vi "Drive Initialize.vi"(8 "Right Slave":u8, 9 "Right Master":u8, 10 "Left Slave":u8, 11 "Left Master":u8) -> (1 "RightMasterDevRef":T1, 3 "LeftMasterDevRef":T1)   [LabVIEW 2019]
uses:
  <vilib>/Rock Robotics/WPI/MotorControl/WPI_MotorControlDeviceRef.ctl
  <vilib>/Rock Robotics/WPI/MotorControl/WPI_MotorControlType.ctl
  <vilib>/Rock Robotics/SystemInterfaces/DIO/FPGA_DIOPWMChannel.ctl
  <vilib>/Rock Robotics/WPI/PWM/WPI_PWMDeadband.ctl
  <vilib>/Rock Robotics/SystemInterfaces/DIO/FPGA_DIOChannel.ctl
  <vilib>/Rock Robotics/WPI/ThirdParty/Phoenix-LabVIEW/Motor Controller/Controls/CTRE_Phoenix_MotorControl_NeutralMode.ctl
  .Team Code/Contants.vi
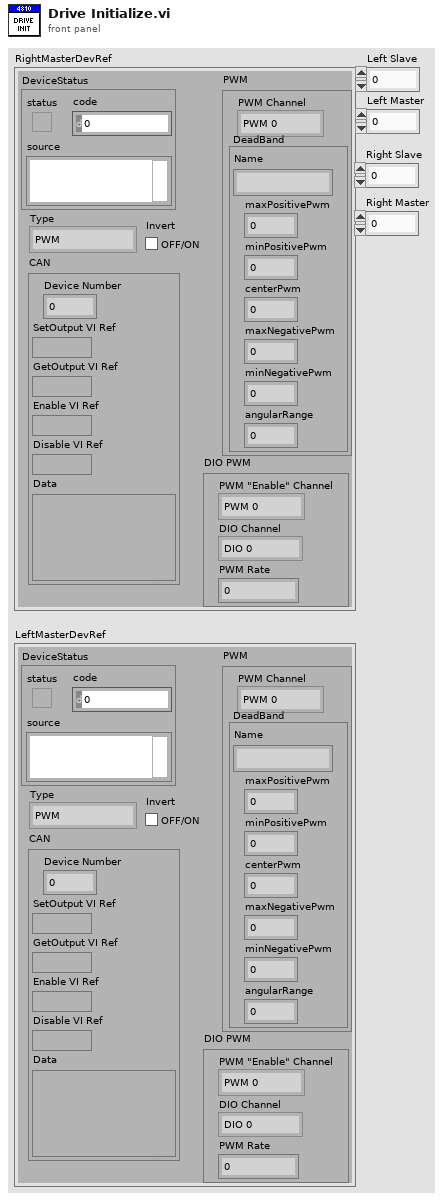
[diagram p1: front panel]
types:
  T1 = typedef "WPI_MotorControlDeviceRef.ctl" = cluster{"DeviceStatus":errorcluster, "Type":T2, "PWM":cluster{"PWM Channel":T3, "DeadBand":T4}, "CAN":cluster{"Device Number":u8, "SetOutput VI Ref":variant, "GetOutput VI Ref":variant, "Enable VI Ref":variant, "Disable VI Ref":variant, "Data":variant}, "Invert":bool, "DIO PWM":cluster{"PWM \"Enable\" Channel":T3, "DIOChannel":T5, "PWM Rate":dbl}}
  T2 = typedef "WPI_MotorControlType.ctl" = enum16{"PWM", "CAN", "DIO PWM"}
  T3 = typedef "FPGA_DIOPWMChannel.ctl" = enum8{"PWM 0", "PWM 1", "PWM 2", "PWM 3", "PWM 4", "PWM 5", "PWM 6", "PWM 7", "PWM 8", "PWM 9", "PWM MXP 0", "PWM MXP 1", "PWM MXP 2", "PWM MXP 3", "PWM MXP 4", "PWM MXP 5", "PWM MXP 6", "PWM MXP 7", "PWM MXP 8", "PWM MXP 9", "Invalid"}
  T4 = typedef "WPI_PWMDeadband.ctl" = cluster{"Name":string, "maxPositivePwm":i32, "minPositivePwm":i32, "centerPwm":i32, "maxNegativePwm":i32, "minNegativePwm":i32, "angularRange":u16}
  T5 = typedef "FPGA_DIOChannel.ctl" = enum8{"DIO 0", "DIO 1", "DIO 2", "DIO 3", "DIO 4", "DIO 5", "DIO 6", "DIO 7", "DIO 8", "DIO 9", "DIO MXP 0", "DIO MXP 1", "DIO MXP 2", "DIO MXP 3", "DIO MXP 4", "DIO MXP 5", "DIO MXP 6", "DIO MXP 7", "DIO MXP 8", "DIO MXP 9", "DIO MXP 10", "DIO MXP 11", "DIO MXP 12", "DIO MXP 13", "DIO MXP 14", "DIO MXP 15", "SPI Port CS1", "SPI Port CS2", "SPI Port CS3", "SPI Port MISO", "SPI Port MOSI", "Invalid"}
  T6 = typedef "CTRE_Phoenix_MotorControl_NeutralMode.ctl" = enum8{"EEPROMSetting", "Override to Coast", "Override to Brake"}
  T7 = cluster{"Cruise Velocity":i32, "Acceleration":i32}
  T8 = cluster{"P":dbl, "I":dbl, "D":dbl, "F":dbl, "I Zone":dbl}
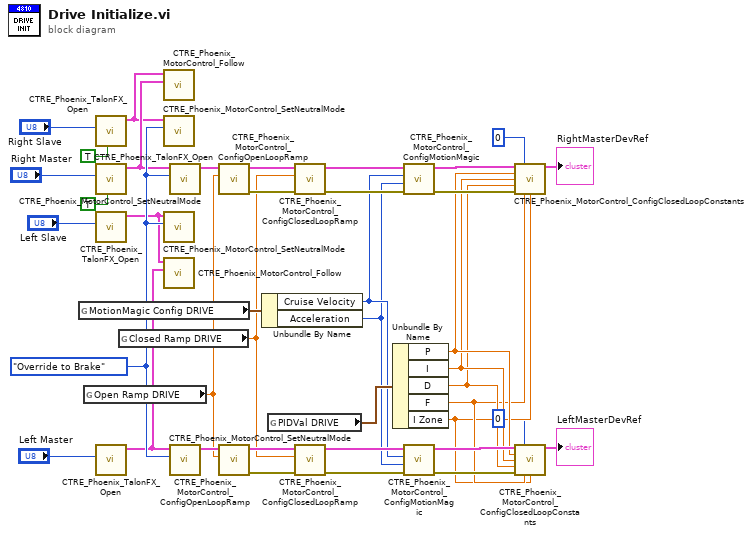
[diagram p0: block diagram]
diagram:
  w40 = CTRE_Phoenix_MotorControl_NeutralMode."Override to Brake" ("Motor Control Neutral Mode")
  n1 = global read "Contants.vi" "MotionMagic Config DRIVE"() -> (w15:T7)
  n2 = global read "Contants.vi" "Open Ramp DRIVE"() -> (w5:dbl)
  n3 = call <vilib>:"CTRE_Phoenix_TalonFX_Open.vi"("Invert"=TRUE, "Device Number"="Right Slave") -> ("CAN Talon SRX Ref"=w38:T1)  [unwired: 8 in, 1 out]
  n4 = call <vilib>:"CTRE_Phoenix_TalonFX_Open.vi"("Invert"=TRUE, "Device Number"="Right Master") -> ("CAN Talon SRX Ref"=w39:T1)  [unwired: 8 in, 1 out]
  n5 = call <vilib>:"CTRE_Phoenix_TalonFX_Open.vi"("Device Number"="Left Slave") -> ("CAN Talon SRX Ref"=w36:T1)  [unwired: 9 in, 1 out]
  n6 = call <vilib>:"CTRE_Phoenix_TalonFX_Open.vi"("Device Number"="Left Master") -> ("CAN Talon SRX Ref"=w37:T1)  [unwired: 9 in, 1 out]
  n7 = global read "Contants.vi" "Closed Ramp DRIVE"() -> (w6:dbl)
  n8 = call <vilib>:"CTRE_Phoenix_MotorControl_Follow.vi"("Master Controller to Follow"=w39, "PhoenixMotorControlDevRef"=w38) -> ()  [unwired: 8 in, 2 out]
  n9 = call <vilib>:"CTRE_Phoenix_MotorControl_SetNeutralMode.vi"("Motor Control Neutral Mode"=w40, "PhoenixMotorControlDevRef"=w38) -> ()  [unwired: 8 in, 2 out]
  n10 = call <vilib>:"CTRE_Phoenix_MotorControl_SetNeutralMode.vi"("Motor Control Neutral Mode"=w40, "PhoenixMotorControlDevRef"=w36) -> ()  [unwired: 8 in, 2 out]
  n11 = call <vilib>:"CTRE_Phoenix_MotorControl_Follow.vi"("Master Controller to Follow"=w37, "PhoenixMotorControlDevRef"=w36) -> ()  [unwired: 8 in, 2 out]
  n12 = call <vilib>:"CTRE_Phoenix_MotorControl_SetNeutralMode.vi"("Motor Control Neutral Mode"=w40, "PhoenixMotorControlDevRef"=w39) -> ("PhoenixMotorControlDevRef"=w17:T1)  [unwired: 8 in, 1 out]
  n13 = call <vilib>:"CTRE_Phoenix_MotorControl_SetNeutralMode.vi"("Motor Control Neutral Mode"=w40, "PhoenixMotorControlDevRef"=w37) -> ("PhoenixMotorControlDevRef"=w25:T1)  [unwired: 8 in, 1 out]
  n14 = call <vilib>:"CTRE_Phoenix_MotorControl_ConfigOpenLoopRamp.vi"("secondsFromNeutralToFull"=w5, "PhoenixMotorControlDevRef"=w17) -> ("error out"=w18:errorcluster, "PhoenixMotorControlDevRef"=w19:T1)  [unwired: 8 in]
  n15 = call <vilib>:"CTRE_Phoenix_MotorControl_ConfigOpenLoopRamp.vi"("secondsFromNeutralToFull"=w5, "PhoenixMotorControlDevRef"=w25) -> ("error out"=w31:errorcluster, "PhoenixMotorControlDevRef"=w30:T1)  [unwired: 8 in]
  n16 = Unbundle By Name(w15) -> ("Cruise Velocity"=w8:i32, "Acceleration"=w7:i32)
  n17 = global read "Contants.vi" "PIDVal DRIVE"() -> (w14:T8)
  n18 = call <vilib>:"CTRE_Phoenix_MotorControl_ConfigClosedLoopRamp.vi"("error in (no error)"=w18, "secondsFromNeutralToFull"=w6, "PhoenixMotorControlDevRef"=w19) -> ("error out"=w23:errorcluster, "PhoenixMotorControlDevRef"=w20:T1)  [unwired: 7 in]
  n19 = call <vilib>:"CTRE_Phoenix_MotorControl_ConfigClosedLoopRamp.vi"("error in (no error)"=w31, "secondsFromNeutralToFull"=w6, "PhoenixMotorControlDevRef"=w30) -> ("error out"=w26:errorcluster, "PhoenixMotorControlDevRef"=w29:T1)  [unwired: 7 in]
  n20 = Unbundle By Name(w14) -> ("P"=w13:dbl, "I"=w12:dbl, "D"=w11:dbl, "F"=w10:dbl, "I Zone"=w9:dbl)
  n21 = call <vilib>:"CTRE_Phoenix_MotorControl_ConfigMotionMagic.vi"("error in (no error)"=w23, "Acceleration"=w7, "Cruise Velocity"=w8, "PhoenixMotorControlDevRef"=w20) -> ("error out"=w22:errorcluster, "PhoenixMotorControlDevRef"=w21:T1)  [unwired: 6 in]
  n22 = call <vilib>:"CTRE_Phoenix_MotorControl_ConfigMotionMagic.vi"("error in (no error)"=w26, "Acceleration"=w7, "Cruise Velocity"=w8, "PhoenixMotorControlDevRef"=w29) -> ("error out"=w27:errorcluster, "PhoenixMotorControlDevRef"=w28:T1)  [unwired: 6 in]
  n23 = call <vilib>:"CTRE_Phoenix_MotorControl_ConfigClosedLoopConstants.vi"("PhoenixMotorControlDevRef"=w21, "slotIdx"=0, "P"=w13, "I"=w12, "D"=w11, "error in (no error)"=w22, "F"=w10, "I Zone"=w9) -> ("PhoenixMotorControlDevRef"=→"RightMasterDevRef":T1)  [unwired: 6 in, 1 out]
  n24 = call <vilib>:"CTRE_Phoenix_MotorControl_ConfigClosedLoopConstants.vi"("PhoenixMotorControlDevRef"=w28, "slotIdx"=0, "P"=w13, "I"=w12, "D"=w11, "error in (no error)"=w27, "F"=w10, "I Zone"=w9) -> ("PhoenixMotorControlDevRef"=→"LeftMasterDevRef":T1)  [unwired: 6 in, 1 out]
